vi "AODScanner.vi"() -> ()   [LabVIEW 2011]
uses:
  <vilib>/userdefined/High Color/nirio_resource_hc.ctl
  AODAcq/AODAcq.lvclass
  <vilib>/DAQmx/write.llb/DAQmx Write (Analog DBL 1Chan 1Samp).vi
  <vilib>/DAQmx/read.llb/DAQmx Read (Analog Wfm 1Chan NSamp).vi
  <vilib>/DAQmx/miscellaneous.llb/DAQmx Fill In Error Info.vi
  <vilib>/Utility/error.llb/Error Cluster From Error Code.vi
  <vilib>/rvi/errors/niLvFpgaAdjustHostInterfaceError.vi
  <vilib>/rvi/interface/nirviReadWriteControl/nirviReadWriteControl.xnode
  FPGA_Control/AODRef.ctl
  FPGA_Control/FPGA Bitfiles/AODControl_FPGATarget_5751Acquire_F1CF9257.lvbitx
  FPGA_Control/AOD Control (FPGA).vi
  NiFpgaLv.dll
panel:
  out "# elements in queue 4":i32
  out "# elements in queue 3":i32
  out "# elements in queue 2":i32
  out "# elements in queue":i32
  out "Waveform Chart":waveform(dbl)(graph)
  out "Ephys":bool
  in  "TraceElements":u32=10000
  out "ScanProgress":dbl(slide) scale=0.0..1.0
  in  "Abort":bool
  out "Progress":dbl(slide) scale=0.0..1.0
  in  "SweepSettings":bool
  in  "stop":bool
  in  "Power":dbl(slide) min=0.0 max=5.0 step=0.1 scale=0.0..2.5
  out "Point Scanning":bool
  out "Volume Scanning":bool
  in  "Tab Control":enum32{"Setup", "Volume", "Traces", "Motion"}(tab)=enum."Volume"
  in  "Ephys":bool
  in  "Motion rate (Hz)":dbl
  in  "ClearPoints":bool
  in  "Recording Settings":T1
  in  "Scan Settings (um)":T2={"XStart"=-100, "XEnd"=100, "XNum"=250, "YStart"=-100, "YEnd"=100, "YNum"=250, "ZStart"=-50, "ZEnd"=50, "ZNum"=30}
  in  "RIO Device":T3="RIO0"
  in  "Objective":enum16{"20x Olympus"}(ring)
  in  "Scan Time (s)":dbl=300.0
  in  "Volume Reps":i32=1 min=1 max=10000
  in  "Volume":bool
  in  "Scan":bool
  in  "Decimate":bool
  out "Motion points":u32
  in  "MaxThreshold":dbl=1.0
  out "Number selected":u32
  in  "Number of cells":u32=200
  in  "Threshold":dbl=0.1
  in  "Max":dbl(slide)=700000.0 scale=0.0..1310720.0
  out "ImCh2":T4(plugin-control)
  out "ImCh1":T4(plugin-control)
  in  "Section":dbl min=0.0 max=29.0 step=1.0
  in  "Segment":bool
  out "Motion Increment":u32
  in  "DisplayVol":bool=TRUE
  out "Motion Ch1":T4(plugin-control)
  out "Ephys":waveform(dbl)[](graph)
  out "Traces":waveform(dbl)[](graph)
  in  "Down Rate":i32=500
  in  "Spacing":dbl=100.0
  out "Motion Ch2":T4(plugin-control)
  out "Finished":bool
  out "Stopped":bool
  out "AODAcq out":refnum<class "AODAcq.lvclass">
  in  "Debug":bool
  in  "GridPoints":u16=10
  out "Scan Settings":T2
  out "VolData":u8[][](array[numeric])
  in  "VolumeElements":u32=10000
  in  "Points":i32[][](array[numeric])
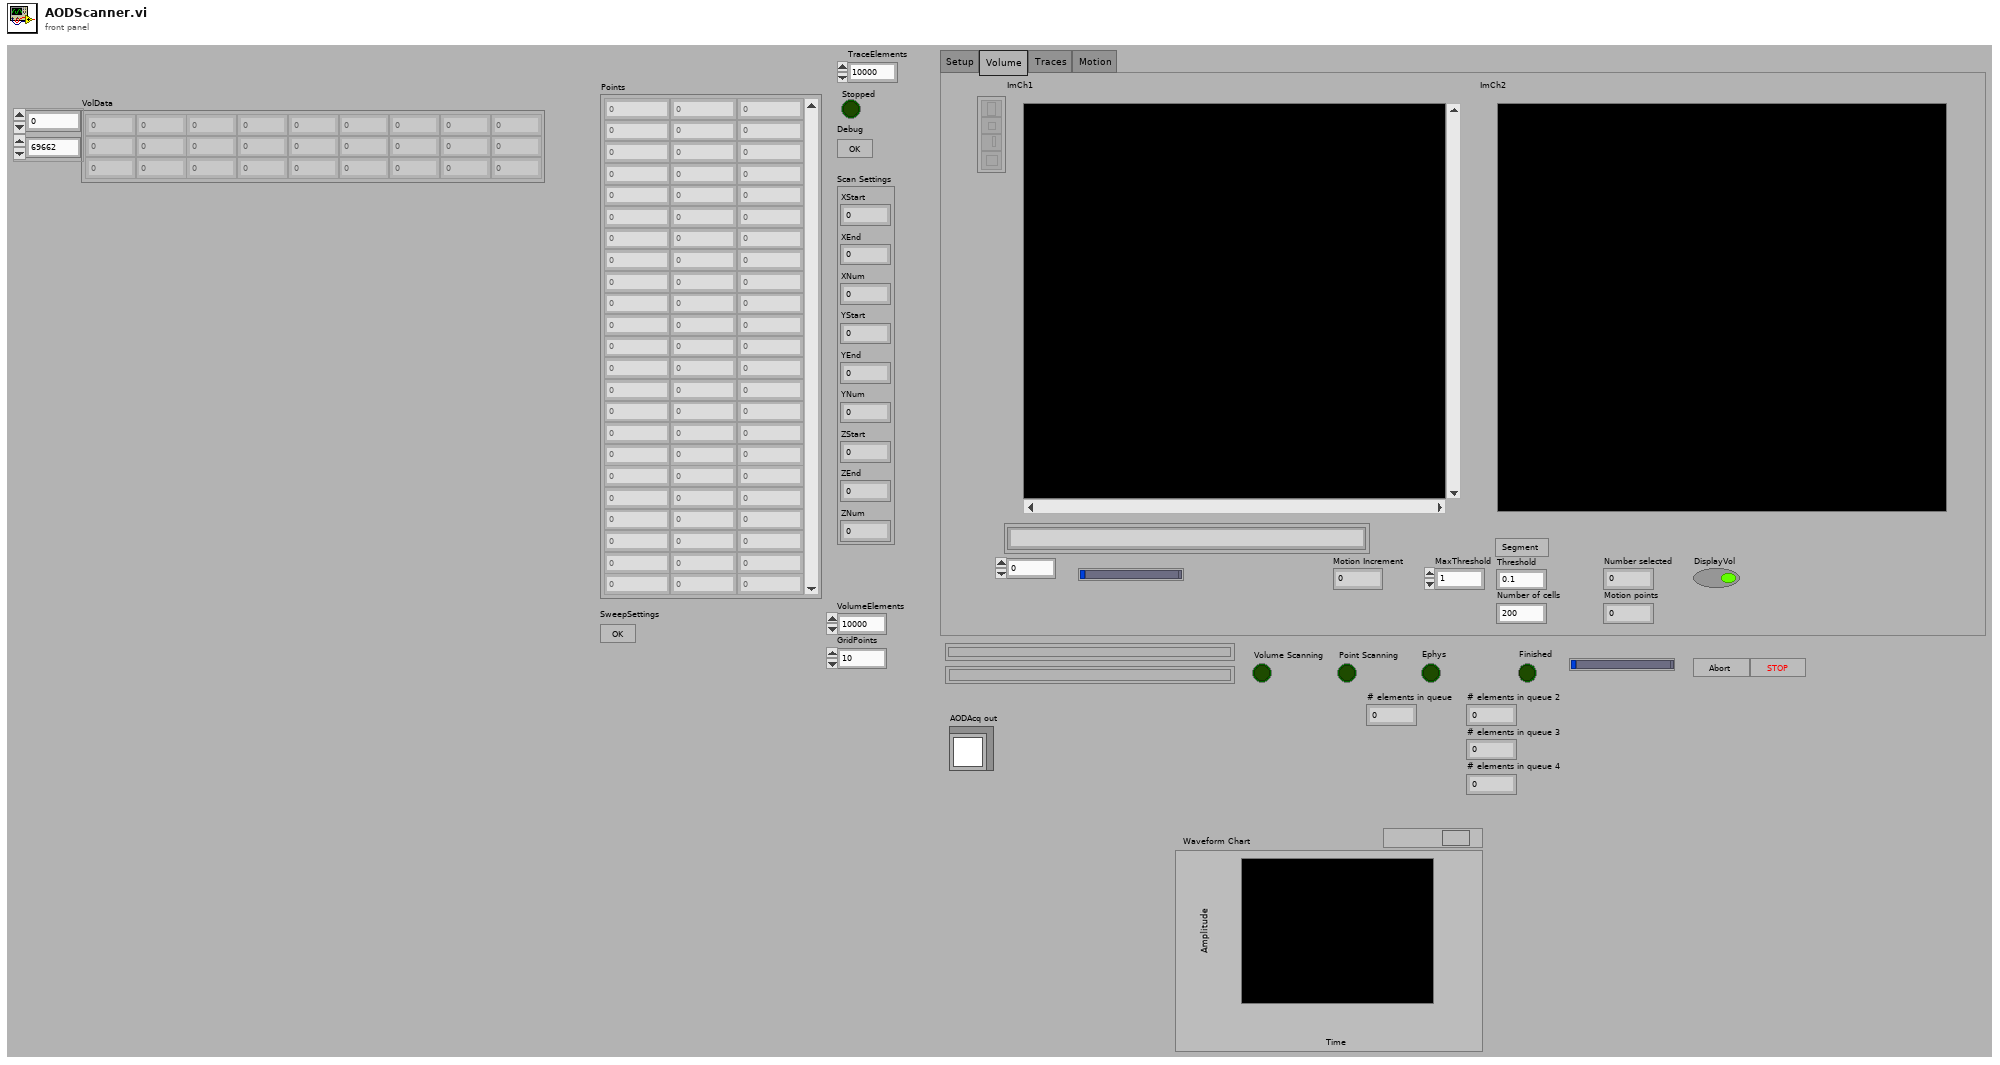
[diagram p1: front panel]
types:
  T1 = cluster{"Path":path, "Save":bool, "SaveRaw":bool}
  T2 = cluster{"XStart":i32, "XEnd":i32, "XNum":i32, "YStart":i32, "YEnd":i32, "YNum":i32, "ZStart":i32, "ZEnd":i32, "ZNum":i32}
  T3 = typedef "nirio_resource_hc.ctl" = tag
  T4 = typedef "IMAQ Image.ctl" = refnum<image>
  T5 = typedef "Image Type" = u32
  T6 = cluster{"Global Rectangle":i32[], "Contours":cluster{"Contour Type":u32, "ROI Type":u32, "Points":i32[]}[]}
  T7 = cluster{"queue out":refnum<queue>, "queue out":refnum<queue>, "queue out":refnum<queue>}
  T8 = typedef "AODRef.ctl" = refnum<k20>
  T9 = cluster{"Global Rectangle":i32[], "Contours":cluster{"Contour Type":u32, "ROI Type":u32, "Points":i32[]}[]}[]
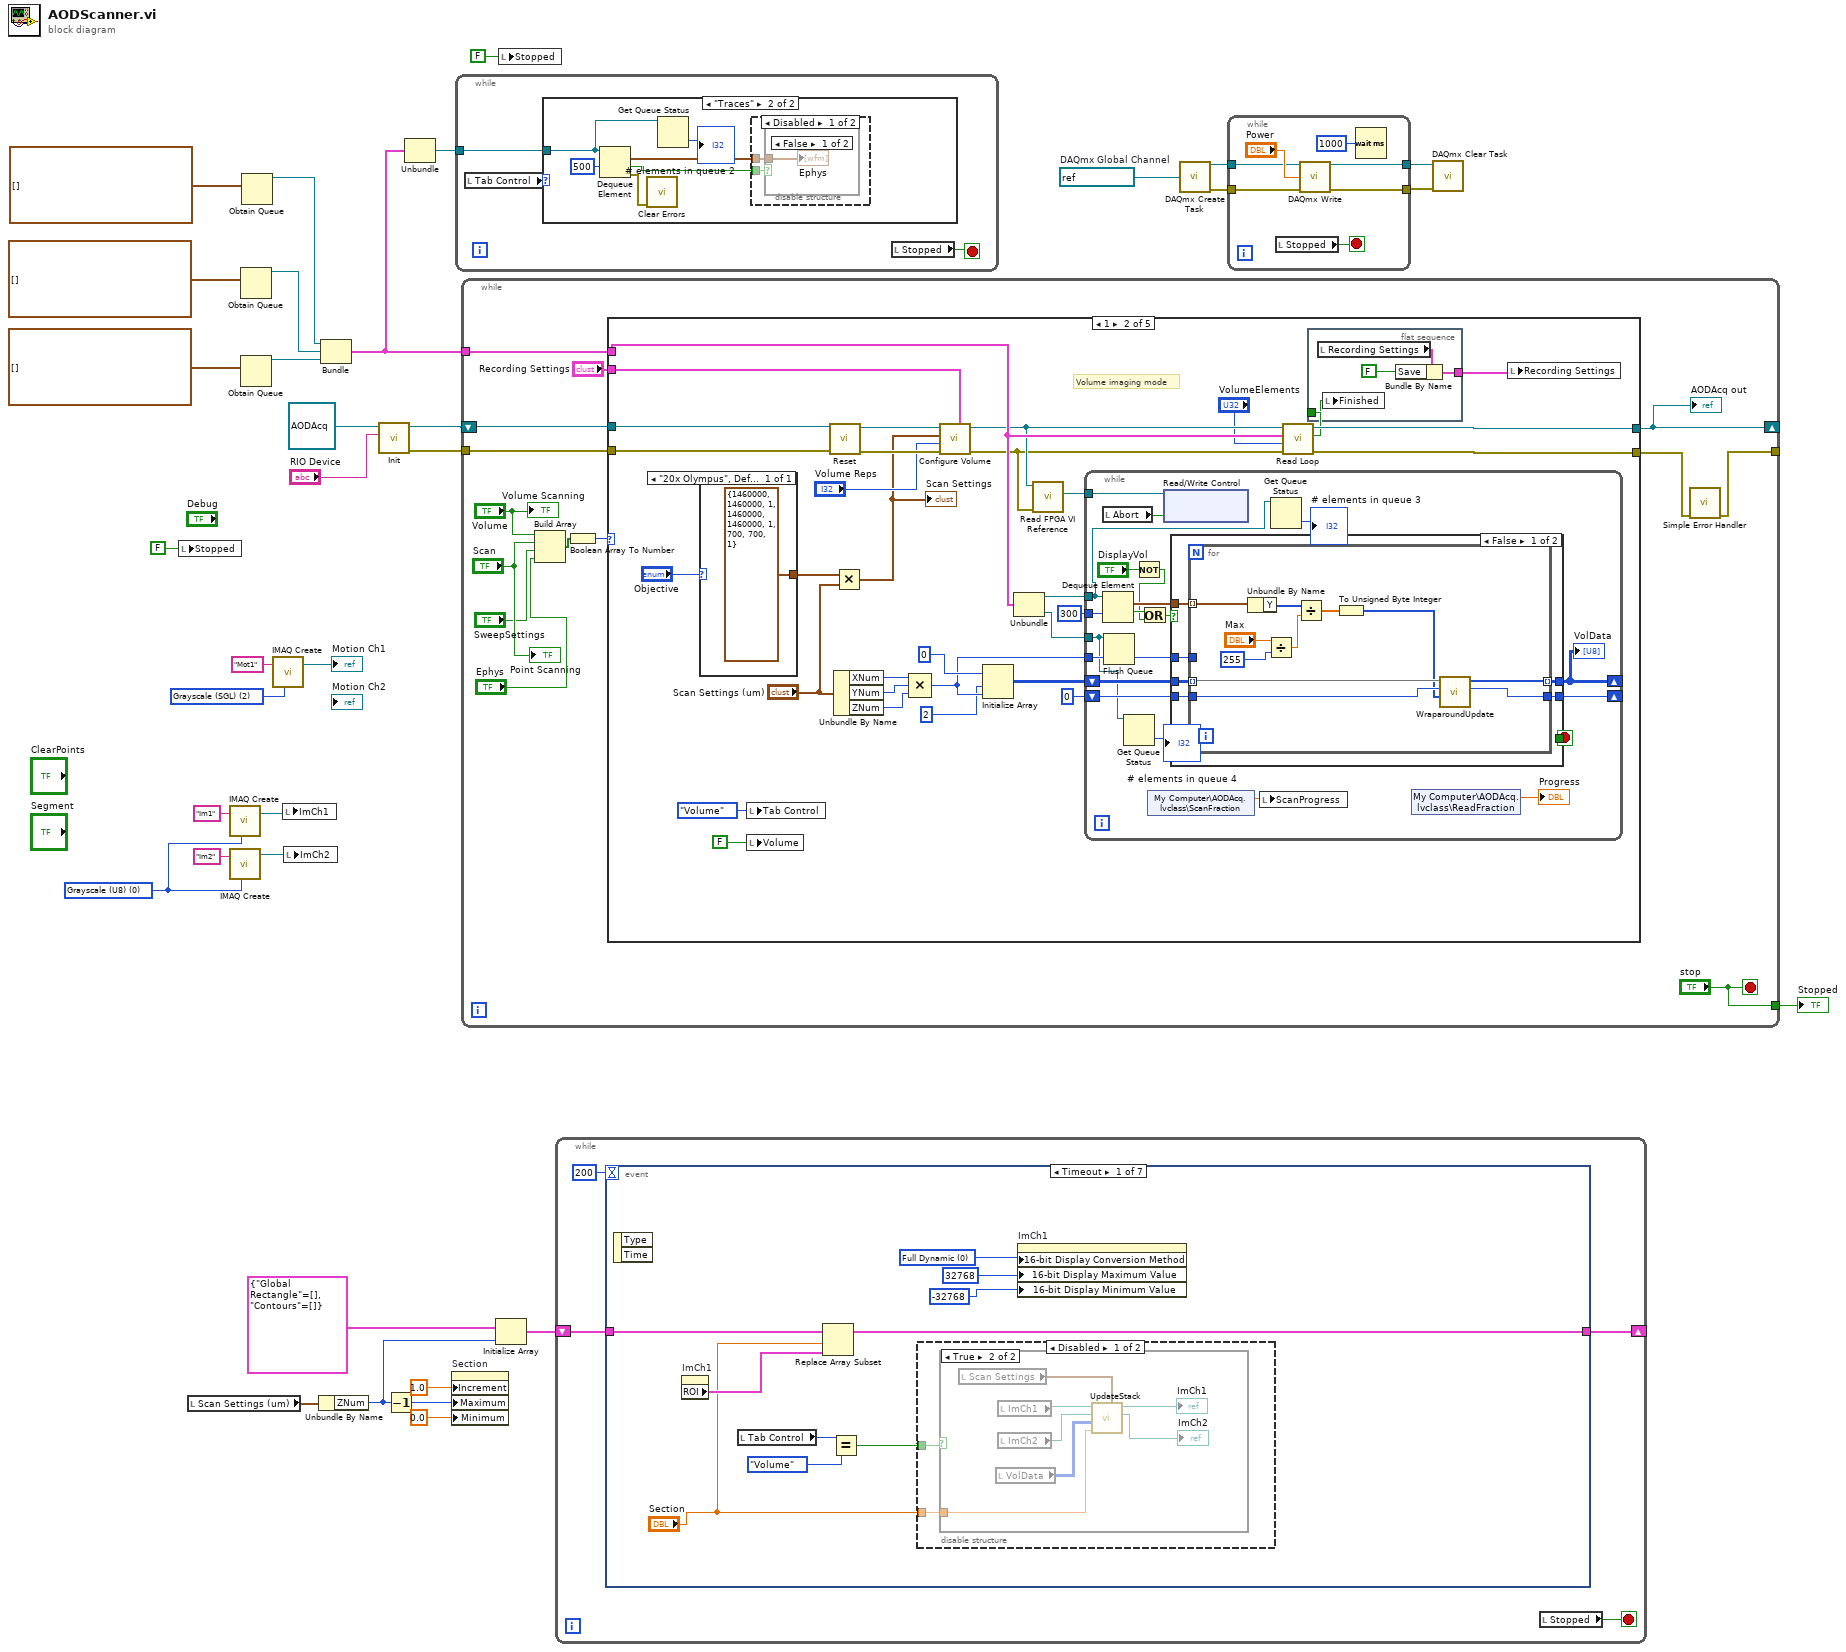
[diagram p0: block diagram]
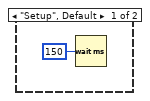
[diagram p2: hidden frame]
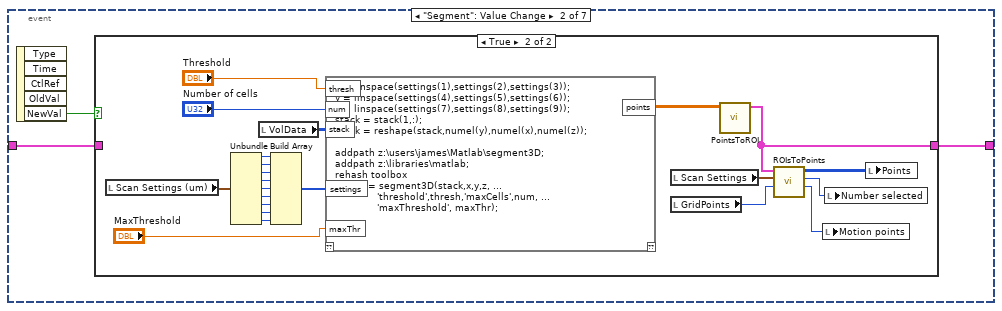
[diagram p7: hidden frame]
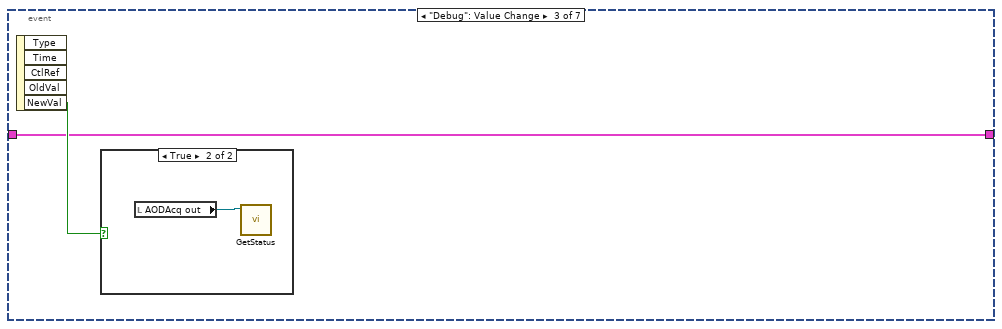
[diagram p9: hidden frame]
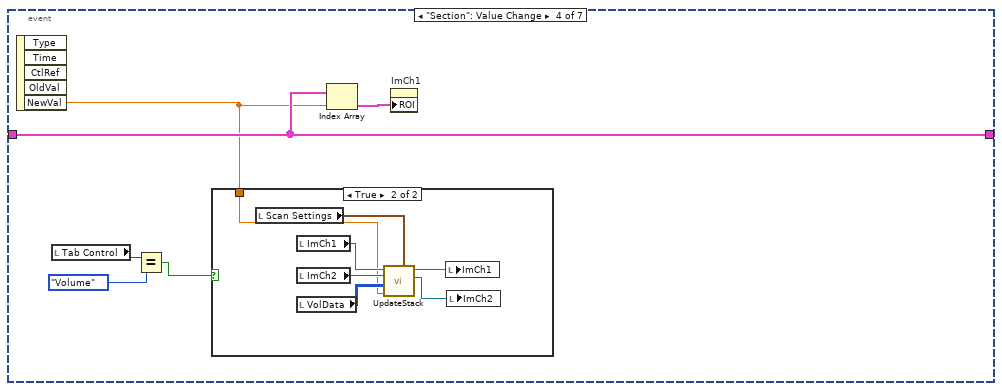
[diagram p11: hidden frame]
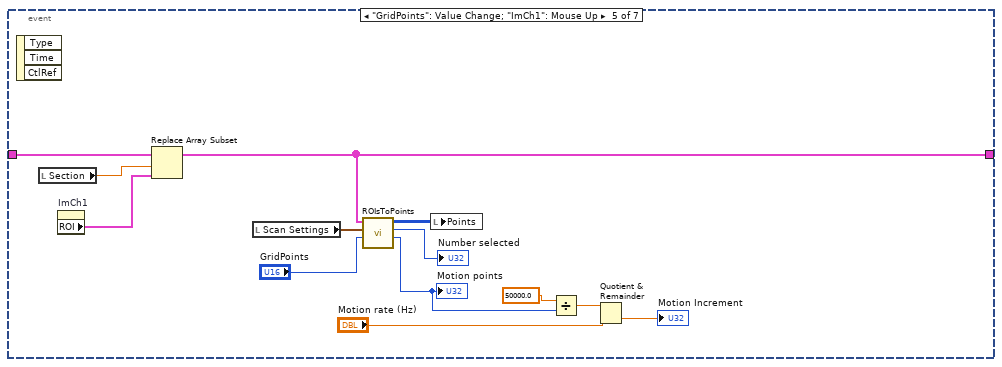
[diagram p13: hidden frame]
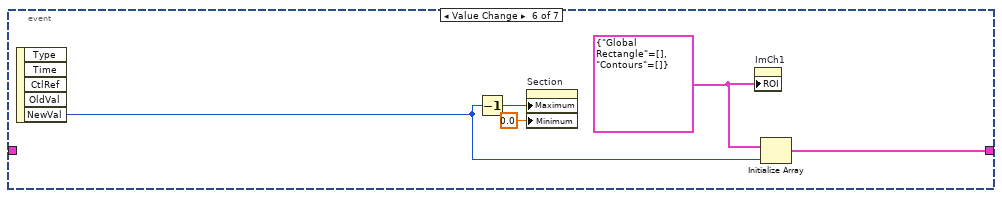
[diagram p14: hidden frame]
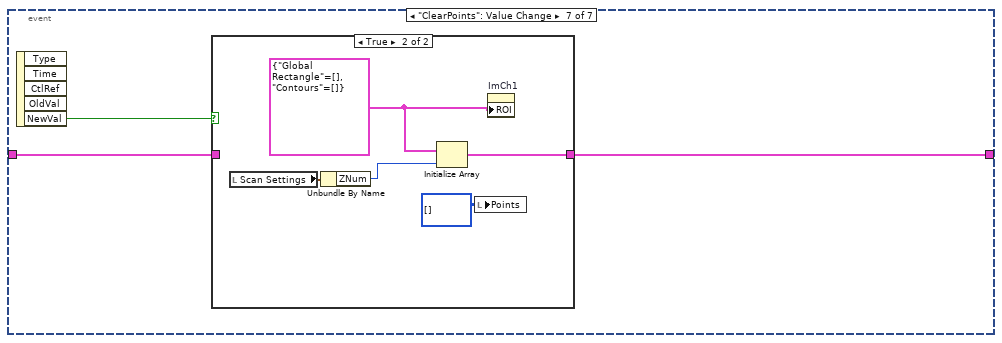
[diagram p15: hidden frame]
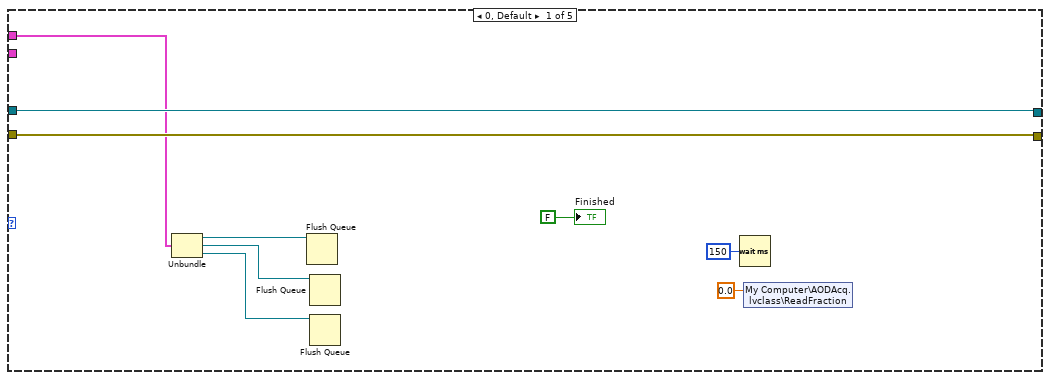
[diagram p17: hidden frame]
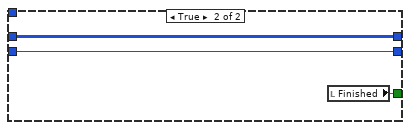
[diagram p18: hidden frame]
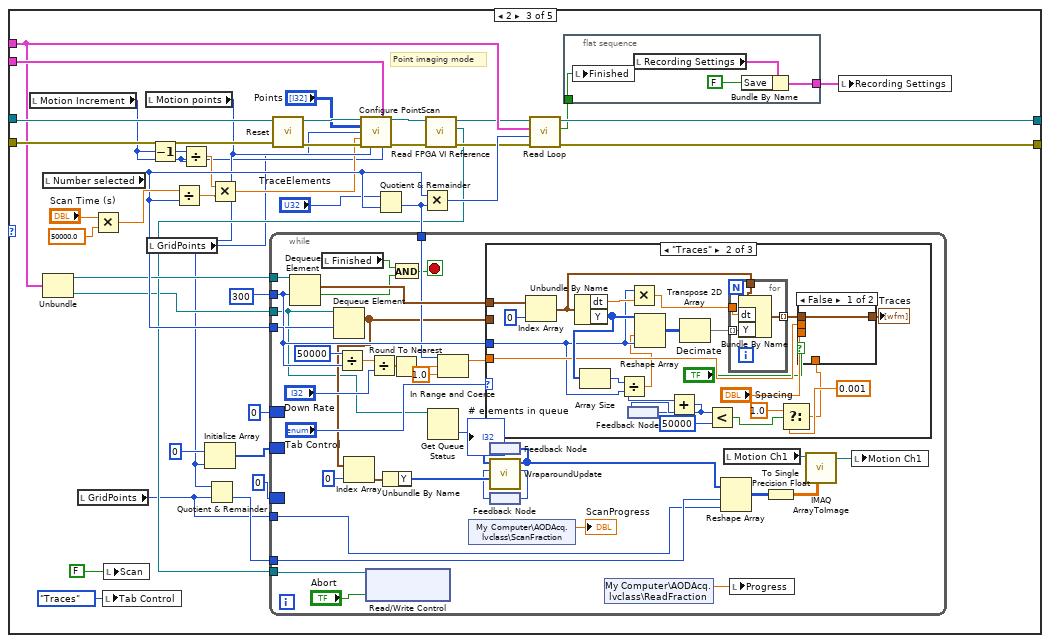
[diagram p19: hidden frame]
diagram:
  w2 = T5 2 items=["Grayscale (U8)", "Grayscale (I16)", "Grayscale (SGL)", "Complex (CSG)", "RGB (U32)", "HSL (U32)", "RGB (U64)", "Grayscale (U16)"] ("Image Type")
  w14 = T5 0 items=["Grayscale (U8)", "Grayscale (I16)", "Grayscale (SGL)", "Complex (CSG)", "RGB (U32)", "HSL (U32)", "RGB (U64)", "Grayscale (U16)"] ("Image Type")
  w26 = refnum<k21> "AOD Gain"  # DAQmx Global Channel
  n1 = local write "Stopped"(FALSE ("Stopped")) -> ()
  n2 = local read "Scan Settings (um)"() -> (w19:T2)
  n3 = call "IMAQ Create"("Image Name"="Im1", "Image Type"=w14) -> ("New Image"=w28:T4)  [unwired: 3 in, 1 out]
  n4 = call "IMAQ Create"("Image Name"="Im2", "Image Type"=w14) -> ("New Image"=w27:T4)  [unwired: 3 in, 1 out]
  n5 = Obtain Queue(element data type=waveform(dbl)[] []) -> (queue out=w9:refnum<queue>)  [unwired: 4 in, 2 out]
  n6 = Obtain Queue(element data type=waveform(i32)[] []) -> (queue out=w7:refnum<queue>)  [unwired: 4 in, 2 out]
  n7 = Obtain Queue(element data type=waveform(i32)[] []) -> (queue out=w8:refnum<queue>)  [unwired: 4 in, 2 out]
  n8 = call "IMAQ Create"("Image Name"="Mot1", "Image Type"=w2) -> ("New Image"=→"Motion Ch1":T4)  [unwired: 3 in, 1 out]
  n9 = local write "ImCh1"(w28) -> ()
  n10 = local write "ImCh2"(w27) -> ()
  n11 = Unbundle By Name(w19) -> ("ZNum"=w13:i32)
  n12 = Bundle("queue out"=w8, "queue out"=w9, "queue out"=w7) -> (w6:T7)  [unwired: 1 in]
  n13 = call "Init.vi"("RIO Device"="RIO Device", "AODAcq in"=refnum<class "AODAcq.lvclass"> refnum ("AODAcq.lvclass")) -> ("error out"=w32:errorcluster, "AODAcq out"=w33:refnum<class "AODAcq.lvclass">)  [unwired: 8 in]
  n14 = Decrement(x=w13) -> (x-1=w12:i32)
  n15 = Unbundle(w6) -> ("queue out"=w5:refnum<queue>)  [unwired: 2 out]
  n16 = property on="Section" class="DigNum (strict)"("Increment"=1.0 ("Data Entry Limits:Increment"), "Maximum"=w12, "Minimum"=0.0 ("Data Entry Limits:Minimum")) -> ()  [unwired: 2 in, 2 out]
  n17 = while {
    tunnel: w5 -> [w38]
    stop <- w37 stop-if-true
    n18 = local read "Tab Control"() -> (w36:enum32{"Setup", "Volume", "Traces", "Motion"})
    n19 = case shown="\"Traces\"" w36 {
      tunnel: w38 -> [_ w41]
      frame "Setup", Default {
        n20 = Wait (ms)(milliseconds to wait=u32 150) -> ()  [unwired: 1 out]
      }
      frame "Traces" {
        n21 = Dequeue Element(queue=w41, timeout in ms (-1)=500) -> (element=w43:waveform(dbl)[], timed out?=w42:bool, error out=w44:errorcluster)  [unwired: 1 in, 1 out]
        n22 = call <vilib>:"Clear Errors.vi"("error in (no error)"=w44) -> ()  [unwired: 6 in, 1 out]
        n23 = Get Queue Status(queue=w41) -> (# elements in queue=→"# elements in queue 2":i32)  [unwired: 2 in, 7 out]
        n24 = disable-structure shown="Disabled" {
          disable-tunnel: w43 -> [w47 _]
          disable-tunnel: w42 -> [w46 _]
          frame Disabled {
            n25 = case shown="False" w46 {
              tunnel: w47 -> [w48 _]
              frame False {
                "Ephys" <- w48
              }
              frame True {
              }
            }
          }
          frame Enabled {
          }
        }
      }
    }
    n26 = local read "Stopped"() -> (w37:bool)
  }
  n27 = while {
    shift-right: [w54] -> _
    shift-left: w33 -> [w62]
    tunnel: w6 -> [w56]
    tunnel: w32 -> [w61]
    tunnel: [w52] -> _
    tunnel: ["stop"] -> w23
    stop <- "stop" stop-if-true
    n28 = Build Array("Volume", "Scan", "SweepSettings", "Ephys") -> (w58:bool[])
    n29 = Boolean Array To Number(Boolean array=w58) -> (number=w57:u32)
    n30 = case shown="1" w57 {
      tunnel: w62 -> [w67 w103 w189 w266 w289]
      tunnel: w61 -> [w70 w102 w188 w265 _]
      tunnel: [w67 w82 w174 w270 w289] -> w54
      tunnel: [w70 w81 w173 w269 w288] -> w53
      tunnel: w56 -> [w66 w80 w172 _ w291]
      tunnel: "Recording Settings" -> [_ w96 w185 _ _]
      frame 0, Default {
        n31 = Unbundle(w66) -> ("queue out"=w65:refnum<queue>, "queue out"=w64:refnum<queue>, "queue out"=w63:refnum<queue>)
        n32 = Flush Queue(queue=w65) -> ()  [unwired: 1 in, 3 out]
        n33 = Flush Queue(queue=w64) -> ()  [unwired: 1 in, 3 out]
        n34 = Flush Queue(queue=w63) -> ()  [unwired: 1 in, 3 out]
        n35 = Wait (ms)(milliseconds to wait=u32 150) -> ()  [unwired: 1 out]
        n36 = shared-variable "My Computer\\AODAcq.lvclass\\ReadFraction"(0.0 ("ReadFraction")) -> ()  [unwired: 1 in, 1 out]
        "Finished" <- FALSE ("Finished")
      }
      frame 1 {
        # "Volume imaging mode"
        n37 = case shown="\"20x Olympus\", Default" "Objective" {
          tunnel: [T2 {"XStart"=1460000, "XEnd"=1460000, "XNum"=1, "YStart"=1460000, "YEnd"=1460000, "YNum"=1, "ZStart"=700, "ZEnd"=700, "ZNum"=1} ("y")] -> w92
          frame "20x Olympus", Default {
          }
        }
        n38 = local write "Tab Control"(enum32{"Setup", "Volume", "Traces"}."Volume" ("Tab Control")) -> ()
        n39 = local write "Volume"(FALSE ("Volume")) -> ()
        n40 = call-dynamic "Reset.vi"("error in (no error)"=w102, "AODAcq in"=w103) -> ("error out"=w100:errorcluster, "AODAcq out"=w101:refnum<class "AODAcq.lvclass">)  [unwired: 8 in]
        n41 = Multiply(x=w92, y="Scan Settings (um)") -> (x*y=w97:T2)
        "Scan Settings" <- w97
        n42 = Unbundle By Name("Scan Settings (um)") -> ("XNum"=w95:i32, "YNum"=w94:i32, "ZNum"=w93:i32)
        n43 = Compound Arithmetic op=MULTIPLY(w95, w94, w93) -> (w85:i32)
        n44 = call-dynamic "Configure Volume.vi"("Recording Settings"=w96, "error in (no error)"=w100, "NumReps"="Volume Reps", "Scan Settings"=w97, "AODAcq in"=w101) -> ("error out"=w76:errorcluster, "AODAcq out"=w77:refnum<class "AODAcq.lvclass">)  [unwired: 5 in]
        n45 = Initialize Array(u8 0, 2 ("dimension size"), w85) -> (w90:u8[][])
        n46 = Unbundle(w80) -> ("queue out"=w79:refnum<queue>, "queue out"=w72:refnum<queue>)  [unwired: 1 out]
        n47 = call-dynamic "Read FPGA VI Reference.vi"("error in (no error)"=w76, "AODAcq in"=w77) -> ("FPGA VI Reference"=w75:T8)  [unwired: 7 in, 2 out]
        n48 = while {
          tunnel: w79 -> [w111]
          shift-right: [w123] -> _
          shift-left: w90 -> [w127]
          shift-right: [w124] -> _
          shift-left: 0 -> [w125]
          tunnel: w85 -> [w122]
          tunnel: 300 ("timeout in ms (-1)") -> [w121]
          tunnel: w75 -> [w118]
          tunnel: w72 -> [w109]
          stop <- w119 stop-if-true
          n49 = local read "Abort"() -> (w114:bool)
          n50 = Dequeue Element(queue=w111, timeout in ms (-1)=w121) -> (element=w126:waveform(i32)[], timed out?=w116:bool)  [unwired: 1 in, 2 out]
          n51 = Flush Queue(queue=w109) -> ()  [unwired: 1 in, 3 out]
          n52 = Get Queue Status(queue=w109) -> (# elements in queue=→"# elements in queue 4":i32)  [unwired: 2 in, 7 out]
          n53 = Not(x="DisplayVol") -> (.not. x?=w112:bool)
          n54 = Or(x=w116, y=w112) -> (x .or. y?=w115:bool)
          n55 = shared-variable "My Computer\\AODAcq.lvclass\\ScanFraction"() -> (w117:dbl)  [unwired: 1 in, 1 out]
          n56 = xnode "Read/Write Control"("FPGA VI Reference In"=w118, "Control.Abort"=w114) -> ()  [unwired: 1 in, 2 out]
          n57 = case shown="False" w115 {
            tunnel: w127 -> [w133 w147]
            tunnel: w126 -> [w132 _]
            tunnel: w125 -> [w131 w146]
            tunnel: [w130 w146] -> w124
            tunnel: [w129 w147] -> w123
            tunnel: w122 -> [w128 _]
            tunnel: [_ w145] -> w119
            frame False {
              n58 = for {
                tunnel: w133 -> [w137] mode=indexing
                tunnel: w132 -> [w144] mode=indexing
                tunnel: [w138] -> w129 mode=indexing
                tunnel: w131 -> [w135]
                tunnel: [w136] -> w130
                tunnel: w128 -> [_]
                n59 = Unbundle By Name(w144) -> ("Y"=w139:i32[])
                n60 = Divide(x="Max", y=255) -> (x/y=w141:dbl)
                n61 = Divide(x=w139, y=w141) -> (x/y=w140:dbl[])
                n62 = To Unsigned Byte Integer(number=w140) -> (unsigned 8bit integer=w134:u8[])
                n63 = call "WraparoundUpdate.vi"("Data"=w134, "Location"=w135, "Accumulator"=w137) -> ("NewLocation"=w136:u32, "Accumulated"=w138:i32[])  [unwired: 7 in]
              }
            }
            frame True {
              n64 = local read "Finished"() -> (w145:bool)
            }
          }
          "VolData" <- w123
          n65 = local write "ScanProgress"(w117) -> ()
          n66 = Get Queue Status(queue=w111) -> (# elements in queue=→"# elements in queue 3":i32)  [unwired: 2 in, 7 out]
          n67 = shared-variable "My Computer\\AODAcq.lvclass\\ReadFraction"() -> (→"Progress":dbl)  [unwired: 1 in, 1 out]
        }
        n68 = call-dynamic "Read Loop.vi"("error in (no error)"=w76, "ReadElements"="VolumeElements", "Queues"=w80, "AODAcq in"=w77) -> ("error out"=w81:errorcluster, "Done"=w78:bool, "AODAcq out"=w82:refnum<class "AODAcq.lvclass">)  [unwired: 5 in]
        n69 = flat-sequence {
          tunnel: w78 -> [w105]
          tunnel: [w104] -> w74
          frame #0 {
            n70 = local read "Recording Settings"() -> (w107:T1)
            n71 = local write "Finished"(w105) -> ()
            n72 = Bundle By Name(cluster=w107, "Save"=FALSE) -> (w104:T1)
          }
        }
        n73 = local write "Recording Settings"(w74) -> ()
      }
      frame 2 {
        # "Point imaging mode"
        n74 = local read "Motion Increment"() -> (w150:u32)
        n75 = local read "Number selected"() -> (w176:u32)
        n76 = Unbundle(w172) -> ("queue out"=w171:refnum<queue>, "queue out"=w164:refnum<queue>)  [unwired: 1 out]
        n77 = local read "GridPoints"() -> (w162:u16)
        n78 = Multiply(x="Scan Time (s)", y=50000.0) -> (x*y=w181:dbl)
        n79 = local write "Tab Control"(enum32{"Setup", "Volume", "Traces"}."Traces" ("Tab Control")) -> ()
        n80 = local write "Scan"(FALSE ("Scan")) -> ()
        n81 = local read "Motion points"() -> (w159:u32)
        n82 = local read "GridPoints"() -> (w149:u16)
        n83 = Decrement(x=w150) -> (x-1=w152:u32)
        n84 = Divide(x=w181, y=w176) -> (x/y=w154:dbl)
        n85 = Divide(x=w152, y=w150) -> (x/y=w151:dbl)
        n86 = Initialize Array(0 ("element"), w159) -> (w160:i32[])
        n87 = Quotient & Remainder(x=w159, y=w162) -> (floor(x/y)=w163:u32)  [unwired: 1 out]
        n88 = Multiply(x=w151, y=w154) -> (x*y=w153:dbl)
        n89 = call-dynamic "Reset.vi"("error in (no error)"=w188, "AODAcq in"=w189) -> ("error out"=w186:errorcluster, "AODAcq out"=w187:refnum<class "AODAcq.lvclass">)  [unwired: 8 in]
        n90 = call-dynamic "Configure PointScan.vi"("AODAcq in"=w187, "Recording Settings"=w185, "Points"="Points", "GridSize"=w149, "Reps"=w153, "error in (no error)"=w186, "Motion Points"=w159, "Motion Increment"=w150) -> ("AODAcq out"=w168:refnum<class "AODAcq.lvclass">, "error out"=w170:errorcluster)  [unwired: 6 in]
        n91 = Quotient & Remainder(x="TraceElements", y=w176) -> (floor(x/y)=w177:u32)  [unwired: 1 out]
        n92 = Multiply(x=w176, y=w177) -> (x*y=w175:u32)
        n93 = call-dynamic "Read FPGA VI Reference.vi"("error in (no error)"=w170, "AODAcq in"=w168) -> ("error out"=w169:errorcluster, "FPGA VI Reference"=w166:T8, "AODAcq out"=w167:refnum<class "AODAcq.lvclass">)  [unwired: 7 in]
        n94 = while {
          tunnel: w176 -> [w225]
          tunnel: 300 ("timeout in ms (-1)") -> [w212]
          tunnel: w177 -> [w220]
          tunnel: w171 -> [w218]
          tunnel: w166 -> [w217]
          tunnel: w164 -> [w195]
          tunnel: w163 -> [w204]
          tunnel: w162 -> [w203]
          border: w160 -> [_]
          border: 0 -> [_]
          border: 0 -> [_]
          stop <- w215 stop-if-true
          n95 = Dequeue Element(queue=w218, timeout in ms (-1)=w212) -> (element=w229:waveform(i32)[], timed out?=w214:bool)  [unwired: 1 in, 2 out]
          n96 = local read "Finished"() -> (w213:bool)
          n97 = Dequeue Element(queue=w195, timeout in ms (-1)=w212) -> (element=w211:waveform(i32)[])  [unwired: 1 in, 3 out]
          n98 = Divide(x=50000, y=w225) -> (x/y=w224:dbl)
          n99 = Index Array(array=w211, index=0) -> (element=w209:waveform(i32))
          n100 = xnode "Read/Write Control"("FPGA VI Reference In"=w217, "Control.Abort"="Abort") -> ()  [unwired: 1 in, 2 out]
          n101 = Divide(x=w224, y="Down Rate") -> (x/y=w227:dbl)
          n102 = Unbundle By Name(w209) -> ("Y"=w201:i32[])
          n103 = Round To Nearest(number=w227) -> (nearest integer value=w222:dbl)
          n104 = And(x=w213, y=w214) -> (x .and. y?=w215:bool)
          n105 = Get Queue Status(queue=w195) -> (# elements in queue=→"# elements in queue":i32)  [unwired: 2 in, 7 out]
          n106 = In Range and Coerce(upper limit=w220, x=w222, lower limit=1.0) -> (coerced(x)=w219:dbl)  [unwired: 1 out]
          n107 = shared-variable "My Computer\\AODAcq.lvclass\\ScanFraction"() -> (→"ScanProgress":dbl)  [unwired: 1 in, 1 out]
          n108 = case shown="\"Traces\"" "Tab Control" {
            tunnel: w225 -> [_ w242 _]
            tunnel: w229 -> [_ w248 _]
            tunnel: w219 -> [_ w245 _]
            tunnel: w211 -> [_ _ _]
            frame "Setup", Default {
            }
            frame "Traces" {
              n109 = Index Array(array=w248, index=0) -> (element=w249:waveform(i32))
              n110 = Unbundle By Name(w249) -> ("dt"=w251:dbl, "Y"=w247:i32[])
              n111 = Array Size(array=w247) -> (size(s)=w237:i32)
              n112 = Divide(x=w237, y=w242) -> (x/y=w241:dbl)
              n113 = feedback #1() -> (w236:i32)
              n114 = Multiply(x=w242, y=w251) -> (x*y=w250:dbl)
              n115 = Reshape Array(w247, w241, w242) -> (w240:i32[][])
              n116 = Add(x=w237, y=w236) -> (x+y=w232:i32)
              n117 = feedback-in #1(w232) -> ()
              n118 = Transpose 2D Array(2D array=w240) -> (transposed array=w239:i32[][])
              n119 = Less?(x=w232, y=50000) -> (x < y?=w230:bool)
              n120 = for {
                tunnel: w250 -> [w262]
                tunnel: w249 -> [w261]
                tunnel: [w260] -> w244 mode=indexing
                tunnel: w239 -> [w259] mode=indexing
                n121 = Bundle By Name(cluster=w261, "dt"=w262, "Y"=w259) -> (w260:waveform(i32))
              }
              n122 = Select(t=1.0, s=w230, f=0.001 ("Baseline Rate")) -> (s? t:f=w233:dbl)
              n123 = case shown="False" "Decimate" {
                tunnel: "Spacing" -> [_ w258]
                tunnel: w245 -> [_ w257]
                tunnel: w244 -> [w253 w256]
                tunnel: [w253 w255] -> w243
                tunnel: w233 -> [_ w254]
                frame False {
                }
                frame True {
                  n124 = call "CleanupTraces.vi"("Baseline Rate"=w254, "Spacing"=w258, "decimating factor"=w257, "Traces in"=w256) -> ("Traces out"=w255:waveform(dbl)[])  [unwired: 7 in]
                }
              }
              "Traces" <- w243
            }
            frame "Motion" {
            }
          }
          n125 = feedback #2() -> (w200:i32[])
          n126 = feedback #3() -> (w198:u32)
          n127 = call "WraparoundUpdate.vi"("Data"=w201, "Location"=w198, "Accumulator"=w200) -> ("NewLocation"=w199:u32, "Accumulated"=w197:i32[])  [unwired: 7 in]
          n128 = feedback-in #2(w197) -> ()
          n129 = feedback-in #3(w199) -> ()
          n130 = shared-variable "My Computer\\AODAcq.lvclass\\ReadFraction"() -> (w205:dbl)  [unwired: 1 in, 1 out]
          n131 = Reshape Array(w197, w204, w203) -> (w207:i32[][])
          n132 = local read "Motion Ch1"() -> (w206:T4)
          n133 = local write "Progress"(w205) -> ()
          n134 = To Single Precision Float(number=w207) -> (single precision float=w202:sgl[][])
          n135 = call "IMAQ ArrayToImage"("Image Pixels (Float)"=w202, "Image"=w206) -> ("Image Out"=w208:T4)  [unwired: 8 in, 1 out]
          n136 = local write "Motion Ch1"(w208) -> ()
        }
        n137 = call-dynamic "Read Loop.vi"("error in (no error)"=w169, "ReadElements"=w175, "Queues"=w172, "AODAcq in"=w167) -> ("error out"=w173:errorcluster, "Done"=w165:bool, "AODAcq out"=w174:refnum<class "AODAcq.lvclass">)  [unwired: 5 in]
        n138 = flat-sequence {
          tunnel: w165 -> [w191]
          tunnel: [w190] -> w157
          frame #0 {
            n139 = local write "Finished"(w191) -> ()
            n140 = local read "Recording Settings"() -> (w192:T1)
            n141 = Bundle By Name(cluster=w192, "Save"=FALSE) -> (w190:T1)
          }
        }
        n142 = local write "Recording Settings"(w157) -> ()
      }
      frame 4 {
        n143 = call-dynamic "Reset.vi"("error in (no error)"=w265, "AODAcq in"=w266) -> ("error out"=w264:errorcluster, "AODAcq out"=w263:refnum<class "AODAcq.lvclass">)  [unwired: 8 in]
        n144 = call-dynamic "Read FPGA VI Reference.vi"("error in (no error)"=w264, "AODAcq in"=w263) -> ("error out"=w272:errorcluster, "FPGA VI Reference"=w273:T8, "AODAcq out"=w271:refnum<class "AODAcq.lvclass">)  [unwired: 7 in]
        n145 = flat-sequence {
          tunnel: w273 -> [w276]
          tunnel: w272 -> [w274]
          tunnel: w271 -> [w275]
          tunnel: [w275] -> w268
          tunnel: [w274] -> w267
          tunnel: [w278] -> w269
          tunnel: [w277] -> w270
          tunnel: w268 -> [w280]
          tunnel: w267 -> [w279]
          frame #0 {
            n146 = call "SweepSettings.vi"("FPGA VI Reference Out"=w276) -> ()  [unwired: 11 in]
          }
          frame #1 {
            n147 = call-dynamic "GetStatus.vi"("error in (no error)"=w279, "AODAcq in"=w280) -> ("error out"=w278:errorcluster, "AODAcq out"=w277:refnum<class "AODAcq.lvclass">)  [unwired: 7 in, 1 out]
          }
        }
      }
      frame 8 {
        n148 = call "DAQ Assistant"() -> ("task out"=w292:refnum<k21>, "error out"=w287:errorcluster)  [unwired: 16 in, 2 out]
        n149 = local write "Tab Control"(enum32{"Setup", "Volume", "Traces", "Motion"}."Traces" ("Tab Control")) -> ()
        n150 = local write "Ephys"(FALSE ("Ephys")) -> ()
        n151 = Unbundle(w291) -> ("queue out"=w285:refnum<queue>)  [unwired: 2 out]
        n152 = while {
          tunnel: w292 -> [w301]
          tunnel: w285 -> [w300]
          tunnel: [w299] -> w290
          tunnel: w287 -> [w298]
          tunnel: [w296] -> w286
          tunnel: [FALSE ("Ephys")] -> w282
          stop <- w302 stop-if-true
          n153 = call-poly <vilib>:"DAQmx Read.vi"("task/channels in"=w301, "error in"=w298) -> ("task out"=w299:refnum<k21>, "data"=w294:waveform(dbl), "error out"=w297:errorcluster)  [unwired: 11 in]
          "Waveform Chart" <- w294
          n154 = Build Array(w294) -> (w293:waveform(dbl)[])
          n155 = local read "Abort"() -> (w302:bool)
          n156 = Enqueue Element(queue=w300, element=w293, error in (no error)=w297) -> (error out=w296:errorcluster)  [unwired: 1 in, 2 out]
        }
        "Ephys" <- w282
        n157 = local write "Ephys"(TRUE ("Ephys")) -> ()
        n158 = call <vilib>:"DAQmx Clear Task.vi"("task in"=w290, "error in"=w286) -> ("error out"=w288:errorcluster)  [unwired: 13 in]
      }
    }
    "AODAcq out" <- w54
    n159 = call <vilib>:"Simple Error Handler.vi"("error in (no error)"=w53) -> ("error out"=w52:errorcluster)  [unwired: 4 in, 4 out]
    "Volume Scanning" <- "Volume"
    "Point Scanning" <- "Scan"
  }
  "Stopped" <- w23
  n160 = Initialize Array(T6 {"Global Rectangle"=[], "Contours"=[]} ("ROI"), w13) -> (w17:T9)
  n161 = local write "Stopped"(FALSE ("Stopped")) -> ()
  n162 = while {
    shift-right: [w305] -> _
    shift-left: w17 -> [w306]
    stop <- w303 stop-if-true
    n163 = event shown="[0] Timeout" {
      selector: _ -> [_ _ _ _ _ _ _]
      dyn-events: _ -> [_ _ _ _ _ _ _]
      timeout: 200 -> [_ _ _ _ _ _ _]
      tunnel: w306 -> [w315 w327 w352 w359 w380 _ w386]
      tunnel: [w316 w326 w352 w359 w377 w385 w387] -> w305
      event Timeout {
        w310 = u32 0 items=["Full Dynamic", "Downshift", "Given Range", "90% Dynamic", "Given Percent Range"] ("16-bit Display Mapping:Conversion Method")
        n164 = event-data() -> ()  [unwired: 1 in, 2 out]
        n165 = property on="ImCh1" class="ImageControl"() -> ("ROI"=w314:T6)  [unwired: 2 in, 2 out]
        n166 = local read "Tab Control"() -> (w313:enum32{"Setup", "Volume", "Traces", "Motion"})
        n167 = Replace Array Subset(array=w315, new element=w314, index="Section") -> (w316:T9)
        n168 = Equal?(x=w313, y=enum32{"Setup", "Volume", "Traces"}."Volume") -> (x = y?=w311:bool)
        n169 = disable-structure shown="Disabled" {
          disable-tunnel: w311 -> [w318 _]
          disable-tunnel: "Section" -> [w317 _]
          frame Disabled {
            n170 = case shown="True" w318 {
              tunnel: w317 -> [_ w319]
              frame False {
              }
              frame True {
                n171 = local read "Scan Settings"() -> (w320:T2)
                n172 = local read "VolData"() -> (w321:u8[][])
                n173 = local read "ImCh1"() -> (w325:T4)
                n174 = local read "ImCh2"() -> (w324:T4)
                n175 = call "UpdateStack.vi"("Scan Settings"=w320, "Section"=w319, "ImData"=w321, "Im2 2"=w324, "Im1 In"=w325) -> ("Im2 Out"=→"ImCh2":T4, "Im1 Out"=→"ImCh1":T4)  [unwired: 5 in]
              }
            }
          }
          frame Enabled {
          }
        }
        n176 = property on="ImCh1" class="ImageControl"("16-bit Display Conversion Method"=w310, "16-bit Display Maximum Value"=32768 ("16-bit Display Mapping:Maximum Value"), "16-bit Display Minimum Value"=-32768 ("16-bit Display Mapping:Maximum Value")) -> ()  [unwired: 2 in, 2 out]
      }
      event "Segment": Value Change {
        n177 = event-data() -> ("NewVal"=w328:bool)  [unwired: 1 in, 4 out]
        n178 = case shown="True" w328 {
          tunnel: w327 -> [w329 _]
          tunnel: [w329 w336] -> w326
          frame False {
          }
          frame True {
            n179 = local read "Scan Settings (um)"() -> (w351:T2)
            n180 = Unbundle(w351) -> ("XStart"=w350:i32, "XEnd"=w349:i32, "XNum"=w348:i32, "YStart"=w347:i32, "YEnd"=w346:i32, "YNum"=w345:i32, "ZStart"=w344:i32, "ZEnd"=w343:i32, "ZNum"=w342:i32)
            n181 = local read "VolData"() -> (w337:u8[][])
            n182 = Build Array(w350, w349, w348, w347, w346, w345, w344, w343, w342) -> (w341:i32[])
            n183 = script code="x = linspace(settings(1),settings(2),settings(3));\ny = linspace(settings(4),settings(5),settings(6));\nz = linspace(settings(7),settings(8),settings(9));\nstack = stack(1,:);\nstack = reshape(stack,numel(y),numel(x),numel(z));\n\naddpath z:\\users\\james\\Matlab\\segment3D;\naddpath z:\\libraries\\matlab;\nrehash toolbox\npoints = segment3D(stack,x,y,z, ...\n              'threshold',thresh,'maxCells',num, ...\n              'maxThreshold', maxThr);"("stack"=w337, "settings"=w341, "num"="Number of cells", "thresh"="Threshold", "maxThr"="MaxThreshold") -> ("points"=w338:cdb[][])  [unwired: 1 in, 1 out]
            n184 = local read "Scan Settings"() -> (w333:T2)
            n185 = local read "GridPoints"() -> (w332:u16)
            n186 = call "PointsToROI.vi"("Points"=w338) -> ("ROIs"=w336:T9)  [unwired: 10 in]
            n187 = call "ROIsToPoints.vi"("GridPoints"=w332, "Scan Settings"=w333, "ROI"=w336) -> ("Number of motion points"=w330:i32, "Number of points"=w334:i32, "Points"=w335:i32[][])  [unwired: 6 in]
            n188 = local write "Motion points"(w330) -> ()
            n189 = local write "Number selected"(w334) -> ()
            n190 = local write "Points"(w335) -> ()
          }
        }
      }
      event "Debug": Value Change {
        n191 = event-data() -> ("NewVal"=w353:bool)  [unwired: 1 in, 4 out]
        n192 = case shown="True" w353 {
          frame False {
          }
          frame True {
            n193 = local read "AODAcq out"() -> (w354:refnum<class "AODAcq.lvclass">)
            n194 = call-dynamic "GetStatus.vi"("AODAcq in"=w354) -> ()  [unwired: 8 in, 3 out]
          }
        }
      }
      event "Section": Value Change {
        n195 = event-data() -> ("NewVal"=w358:dbl)  [unwired: 1 in, 4 out]
        n196 = local read "Tab Control"() -> (w357:enum32{"Setup", "Volume", "Traces", "Motion"})
        n197 = Equal?(x=w357, y=enum32{"Setup", "Volume", "Traces"}."Volume") -> (x = y?=w355:bool)
        n198 = case shown="True" w355 {
          tunnel: w358 -> [_ w362]
          frame False {
          }
          frame True {
            n199 = local read "Scan Settings"() -> (w361:T2)
            n200 = local read "ImCh1"() -> (w365:T4)
            n201 = local read "ImCh2"() -> (w366:T4)
            n202 = local read "VolData"() -> (w367:u8[][])
            n203 = call "UpdateStack.vi"("Scan Settings"=w361, "Section"=w362, "ImData"=w367, "Im2 2"=w366, "Im1 In"=w365) -> ("Im2 Out"=w364:T4, "Im1 Out"=w363:T4)  [unwired: 5 in]
            n204 = local write "ImCh1"(w363) -> ()
            n205 = local write "ImCh2"(w364) -> ()
          }
        }
        n206 = Index Array(array=w359, index=w358) -> (element=w360:T6)
        n207 = property on="ImCh1" class="ImageControl"("ROI"=w360) -> ()  [unwired: 2 in, 2 out]
      }
      event "GridPoints": Value Change; "ImCh1": Mouse Up {
        n208 = event-data() -> ()  [unwired: 1 in, 3 out]
        n209 = local read "Section"() -> (w378:dbl)
        n210 = property on="ImCh1" class="ImageControl"() -> ("ROI"=w379:T6)  [unwired: 2 in, 2 out]
        n211 = Replace Array Subset(array=w380, new element=w379, index=w378) -> (w377:T9)
        n212 = local read "Scan Settings"() -> (w376:T2)
        n213 = call "ROIsToPoints.vi"("GridPoints"="GridPoints", "Scan Settings"=w376, "ROI"=w377) -> ("Number of motion points"=w371:i32, "Number of points"=→"Number selected":i32, "Points"=w374:i32[][])  [unwired: 6 in]
        "Motion points" <- w371
        n214 = local write "Points"(w374) -> ()
        n215 = Divide(x=50000.0, y=w371) -> (x/y=w370:dbl)
        n216 = Quotient & Remainder(x=w370, y="Motion rate (Hz)") -> (floor(x/y)=→"Motion Increment":dbl)  [unwired: 1 out]
      }
      event "Scan Settings (um).ZNum": Value Change {
        w384 = T6 {"Global Rectangle"=[], "Contours"=[]} ("ROI")
        n217 = event-data() -> ("NewVal"=w381:i32)  [unwired: 1 in, 4 out]
        n218 = Decrement(x=w381) -> (x-1=w382:i32)
        n219 = property on="Section" class="DigNum (strict)"("Maximum"=w382, "Minimum"=0.0 ("Data Entry Limits:Minimum")) -> ()  [unwired: 2 in, 2 out]
        n220 = property on="ImCh1" class="ImageControl"("ROI"=w384) -> ()  [unwired: 2 in, 2 out]
        n221 = Initialize Array(w384, w381) -> (w385:T9)
      }
      event "ClearPoints": Value Change {
        n222 = event-data() -> ("NewVal"=w388:bool)  [unwired: 1 in, 4 out]
        n223 = case shown="True" w388 {
          tunnel: [w389 w394] -> w387
          tunnel: w386 -> [w389 _]
          frame False {
          }
          frame True {
            w393 = T6 {"Global Rectangle"=[], "Contours"=[]} ("ROI")
            n224 = local read "Scan Settings"() -> (w392:T2)
            n225 = Unbundle By Name(w392) -> ("ZNum"=w391:i32)
            n226 = Initialize Array(w393, w391) -> (w394:T9)
            n227 = local write "Points"(i32[][] [] ("Points")) -> ()
            n228 = property on="ImCh1" class="ImageControl"("ROI"=w393) -> ()  [unwired: 2 in, 2 out]
          }
        }
      }
    }
    n229 = local read "Stopped"() -> (w303:bool)
  }
  n230 = call <vilib>:"DAQmx Create Task.vi"("global virtual channels"=w26) -> ("task out"=w25:refnum<k21>, "error out"=w24:errorcluster)  [unwired: 4 in, 9 out]
  n231 = while {
    tunnel: w25 -> [w400]
    tunnel: w24 -> [w399]
    tunnel: [w398] -> w22
    tunnel: [w397] -> w21
    stop <- w396 stop-if-true
    n232 = local read "Stopped"() -> (w396:bool)
    n233 = call-poly <vilib>:"DAQmx Write.vi"("task/channels in"=w400, "data"="Power", "error in"=w399) -> ("task out"=w398:refnum<k21>, "error out"=w397:errorcluster)  [unwired: 10 in, 1 out]
    n234 = Wait (ms)(milliseconds to wait=u32 1000) -> ()  [unwired: 1 out]
  }
  n235 = call <vilib>:"DAQmx Clear Task.vi"("task in"=w22, "error in"=w21) -> ()  [unwired: 13 in, 1 out]
